vi "Read.vi"(8 "error in (no error)":errorcluster, 11 "Save as txt in":refnum<class "Save as txt.lvclass">) -> (0 "error out":errorcluster, 1 "Data(UTF8)":string[][](array[string]), 2 "Data":string[][](array[string]), 3 "Save as txt out":refnum<class "Save as txt.lvclass">)   [LabVIEW 2020, in "Save as txt.lvclass"]
uses:
  Save as txt.lvclass
  Saving OO.lvclass
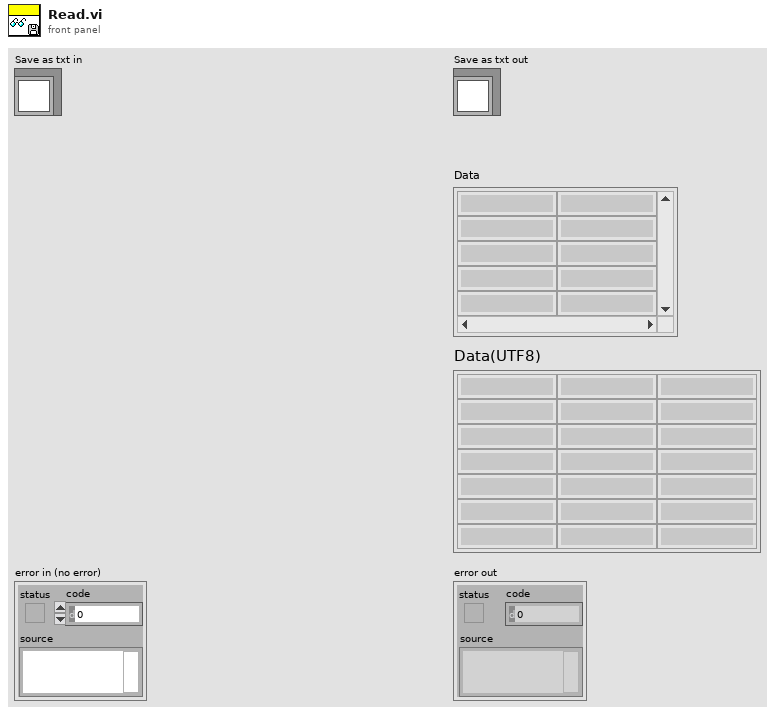
[diagram p1: front panel]
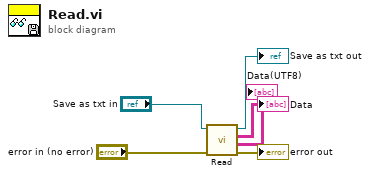
[diagram p0: block diagram]
diagram:
  n1 = call-parent "Read.vi"("error in (no error)"="error in (no error)", "Saving OO in"="Save as txt in") -> ("error out"=→"error out":errorcluster, "Data(UTF8)"=→"Data(UTF8)":string[][], "Data(Text)"=→"Data":string[][], "Saving OO out"=→"Save as txt out":refnum<class "Save as txt.lvclass">)  [unwired: 6 in]
